vi "alarma.vi"(10 "Valor":dbl) -> (1 "Boolean":bool)   [LabVIEW 2018]
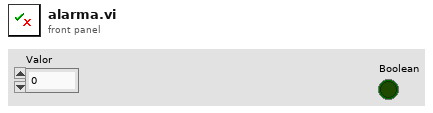
[diagram p1: front panel]
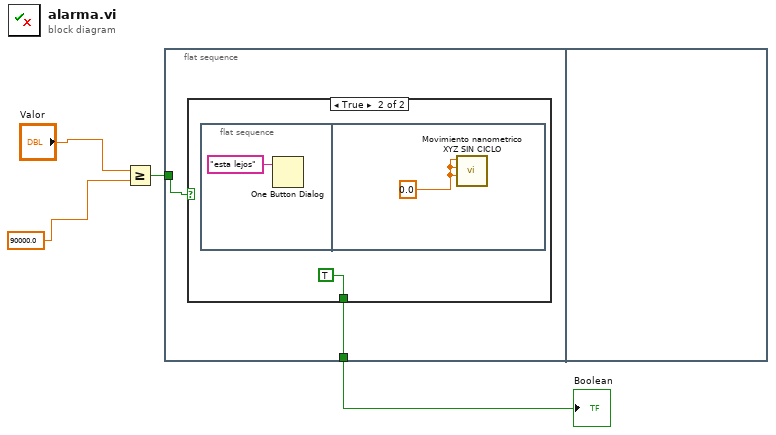
[diagram p0: block diagram]
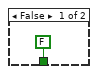
[diagram p2: hidden frame]
diagram:
  n1 = Greater Or Equal?(x="Valor", y=90000.0) -> (x >= y?=w2:bool)
  n2 = flat-sequence {
    tunnel: w2 -> [w6]
    tunnel: [w5] -> w1
    frame #0 {
      n3 = case shown="True" w6 {
        tunnel: [FALSE TRUE] -> w5
        frame False {
        }
        frame True {
          n4 = flat-sequence {
            frame #0 {
              n5 = One Button Dialog(message="esta lejos") -> ()  [unwired: 1 in, 1 out]
            }
            frame #1 {
              w10 = 0.0
              n6 = call "Movimiento nanometrico XYZ SIN CICLO.vi"("Movimiento en Z"=w10, "Movimiento en Y"=w10, "Movimiento en X"=w10) -> ()  [unwired: 3 in, 1 out]
            }
          }
        }
      }
    }
    frame #1 {
    }
  }
  "Boolean" <- w1
